vi "Read Exe Version.vi"(11 "Application name":path=path "INC.exe") -> (0 "Build Date":string, 1 "Application Path out":path, 2 "String":string, 3 "FileVersion":string)   [LabVIEW 2024]
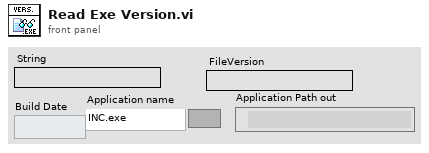
[diagram p1: front panel]
types:
  T1 = enum32{"invalid app kind", "Development System", "Run Time System", "Student Edition", "Embedded LabVIEW", "Evaluation", "Custom"}
  T2 = typedef "FileVersionInformation.ctl" = cluster{"FileVersion":string, "ProductName":string, "InternalName":string, "CompanyName":string, "LegalCopyright":string, "FileDescription":string}
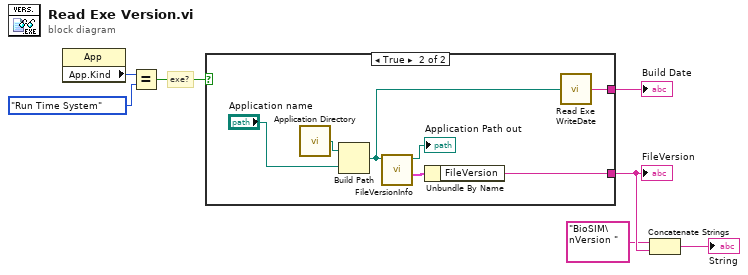
[diagram p0: block diagram]
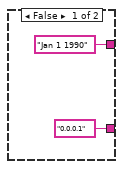
[diagram p2: hidden frame]
diagram:
  # "exe?"
  n1 = property class="App"() -> ("App.Kind"=w4:T1)  [unwired: 2 in, 2 out]
  n2 = Equal?(x=w4, y=T1."Run Time System" ("Application:Kind")) -> (x = y?=w6:bool)
  n3 = case shown="True" w6 {
    tunnel: ["0.0.0.1" ("FileVersion") w15] -> w7
    tunnel: ["Jan 1 1990" ("Last Write Time") w11] -> w1
    frame False {
    }
    frame True {
      n4 = call <vilib>:"Application Directory.vi"() -> ("Application Directory"=w14:path)
      n5 = Build Path(base path=w14, name or relative path="Application name") -> (appended path=w12:path)
      n6 = call <vilib>:"FileVersionInfo.vi"("Application Path in"=w12) -> ("FileVersionInfo Out"=w16:T2, "Application Path out"=→"Application Path out":path)  [unwired: 7 in, 2 out]
      n7 = Unbundle By Name(w16) -> ("FileVersion"=w15:string)
      n8 = call "Read Exe WriteDate.vi"("File Path in"=w12) -> ("Last Write Time"=w11:string)
    }
  }
  "FileVersion" <- w7
  "Build Date" <- w1
  n9 = Concatenate Strings("BioSIM\nVersion " ("Version"), w7) -> (→"String":string)
